vi "Pendulum Write.vi"(9 "motorEffort":i32, 10 "direction":i32, 11 "instance":i32) -> (3 "function return":i32)   [LabVIEW 2025, in "pendulumApp.lvlib"]
doc: "OOTB_API int Pendulum_Write(int instance,int direction,int motorEffort);"
uses:
  pendulumApp.lvlib
  pendulumApp.dll
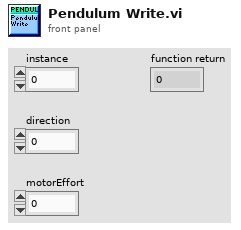
[diagram p1: front panel]
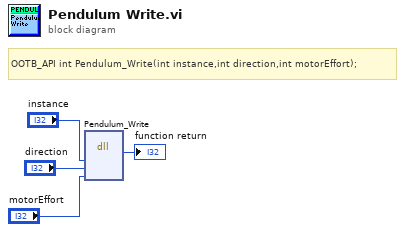
[diagram p0: block diagram]
diagram:
  # "OOTB_API\tint Pendulum_Write(int instance,int direction,int motorEffort);"
  n1 = dll-call lib="C:/Users/noaht/School/Fall 2025/Controls Lab/Lab 3/FA25_pend_Lab3_4/SADI_Pendulum_lib/pendulumApp.*" fn="Pendulum_Write"("instance"="instance", "direction"="direction", "motorEffort"="motorEffort") -> (→"function return":i32)  [unwired: 6 in, 2 out]
